vi "Create DataSet.vi"(8 "error in (no error)":errorcluster caption="错误输入（无错误）", 10 "dataSetName":string, 11 "OleDBClass 输入":refnum<class "OleDBClass.lvclass"> caption="DNL_LabVIEW Object in") -> (0 "error out":errorcluster caption="错误输出", 3 "OleDBClass 输出":refnum<class "OleDBClass.lvclass"> caption="DNL_LabVIEW Object out")   [LabVIEW 2012, in "OleDBClass.lvclass"]
uses:
  OleDBClass.lvclass
  System.Data
  OleDBClass.lvclass/OleDBClass.ctl
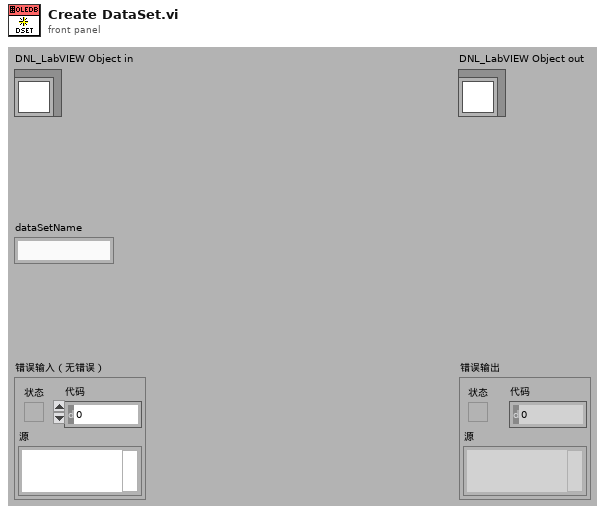
[diagram p1: front panel]
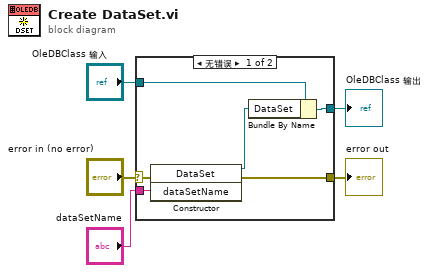
[diagram p0: block diagram]
diagram:
  n1 = case shown="无错误" "error in (no error)" {
    selector: "error in (no error)" -> [w6 w13]
    tunnel: [w7 w13] -> w4
    tunnel: [w8 w12] -> w2
    tunnel: "OleDBClass 输入" -> [w10 w12]
    tunnel: "dataSetName" -> [w11 _]
    frame No Error {
      n2 = constructor class="DataSet"(error in=w6, "dataSetName"=w11) -> (reference out=w9:refnum<k24>, error out=w7:errorcluster)  [unwired: 2 in, 2 out]
      n3 = Bundle By Name(cluster=w10, "DataSet"=w9) -> (w8:refnum<class "OleDBClass.lvclass">)
    }
    frame Error {
    }
  }
  "error out" <- w4
  "OleDBClass 输出" <- w2
